vi "Mono_SetGratingJose.vi"(8 "error in (no error) 2":errorcluster, 9 "Grating":i32, 10 "Mono Wait time (ms)":u32) -> (0 "error out 2":errorcluster, 1 "Wavelength Set":bool=TRUE)   [LabVIEW 2017]
uses:
  C:/Users/Admin/Desktop/Sensitive EQE Stuff/S-EQE (YJ)/Mono vi (YJ)/Cornerstone.dll
  Cornerstone.dll
panel:
  out "CmdLib Out":refnum<k24>
  in  "CmdLib In":refnum<k24>
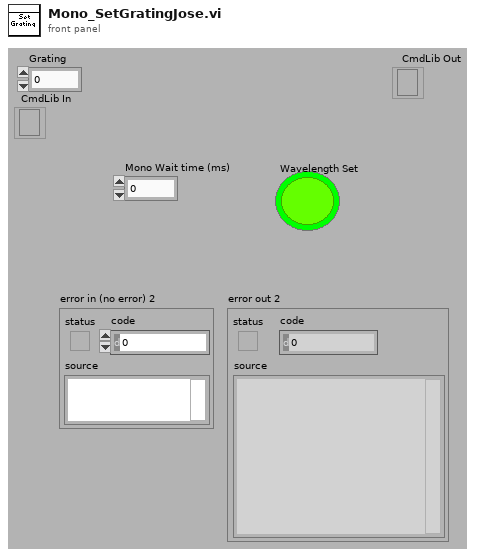
[diagram p1: front panel]
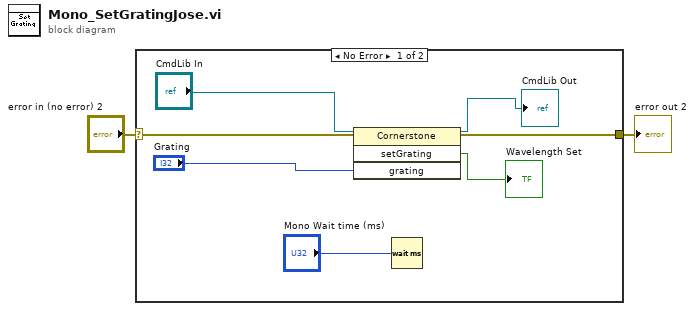
[diagram p0: block diagram]
diagram:
  n1 = case shown="No Error" "error in (no error) 2" {
    selector: "error in (no error) 2" -> [w9 w10]
    tunnel: [w8 w10] -> w1
    frame No Error {
      n2 = invoke class="Cornerstone" method="setGrating"(reference="CmdLib In", error in=w9, "grating"="Grating") -> (reference out=→"CmdLib Out":refnum<k24>, error out=w8:errorcluster, "setGrating"=→"Wavelength Set":bool)  [unwired: 1 in, 1 out]
      n3 = Wait (ms)(milliseconds to wait="Mono Wait time (ms)") -> ()  [unwired: 1 out]
    }
    frame Error {
    }
  }
  "error out 2" <- w1
